vi "Lab5.vi"() -> ()   [LabVIEW 2011]
panel:
  in  "?":bool
  out "Dispersia":dbl
  out "Media":dbl
  out "Suma celor N numere":dbl
  in  "N numere aleatoare":dbl=10.0
  out "Sir care are ultima valoare egala cu Suma numerelor":dbl[](array[numeric]) format="%#.3g"
  out "Sir cu N numere aleatoare":dbl[](array[numeric]) format="%#.3g"
  # "Suma"
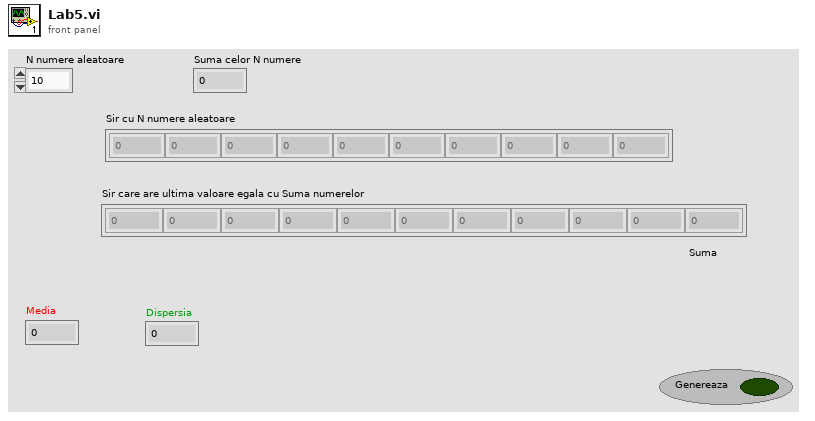
[diagram p1: front panel]
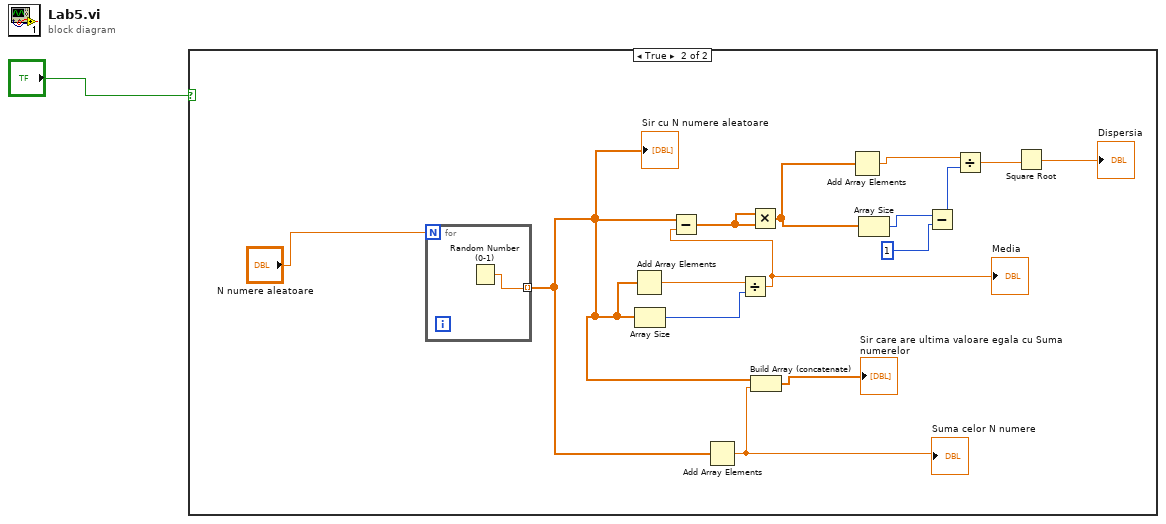
[diagram p0: block diagram]
diagram:
  n1 = case shown="True" "?" {
    frame False {
    }
    frame True {
      n2 = for {
        N: "N numere aleatoare" -> [_]
        tunnel: [w17] -> w10 mode=indexing
        n3 = Random Number (0-1)() -> (number: 0 to 1=w17:dbl)
      }
      "Sir cu N numere aleatoare" <- w10
      n4 = Add Array Elements(numeric array=w10) -> (sum=w15:dbl)
      n5 = Array Size(array=w10) -> (size(s)=w14:i32)
      n6 = Add Array Elements(numeric array=w10) -> (sum=w13:dbl)
      "Suma celor N numere" <- w13
      n7 = Divide(x=w15, y=w14) -> (x/y=w11:dbl)
      "Media" <- w11
      n8 = Subtract(x=w10, y=w11) -> (x-y=w16:dbl[])
      n9 = Multiply(x=w16, y=w16) -> (x*y=w9:dbl[])
      n10 = Build Array (concatenate)(w10, w13) -> (→"Sir care are ultima valoare egala cu Suma numerelor":dbl[])
      n11 = Add Array Elements(numeric array=w9) -> (sum=w5:dbl)
      n12 = Array Size(array=w9) -> (size(s)=w7:i32)
      n13 = Subtract(x=w7, y=1) -> (x-y=w6:i32)
      n14 = Divide(x=w5, y=w6) -> (x/y=w8:dbl)
      n15 = Square Root(x=w8) -> (sqrt(x)=→"Dispersia":dbl)
    }
  }
